vi "StopAcqusition1.vi"(8 "error in (no error)":errorcluster, 11 "Camera_Prime95B in":refnum<class "Camera_Prime95B.lvclass">) -> (0 "error out":errorcluster, 3 "Camera_Prime95B out":refnum<class "Camera_Prime95B.lvclass">)   [LabVIEW 2020]
uses:
  Camera_Prime95B.lvclass
  E:/Development/DevHardSoftware/MicroscopyFramework/Model/Hardware Layer/Real Hardware/Camera_Prime95B/Camera_Prime95B/Dependencies/PVCamNET.dll
  Dependencies/PVCamNET.dll
  Hardware Abstraction Layer/Component/Device/Device/DeviceStatus.ctl
  Hardware Abstraction Layer/Component/Device/Device.lvlib
  E:/Development/DevHardSoftware/MicroscopyFramework/Model/Hardware Abstraction Layer/Component/Camera/Camera/Camera.lvclass
  E:/Development/DevHardSoftware/MicroscopyFramework/Model/Hardware Abstraction Layer/Component/Device/Device/Device.lvclass
  C:/Program Files/National Instruments/LabVIEW 2020/vi.lib/ActorFramework/Actor/Actor.lvclass
  E:/Development/DevHardSoftware/MicroscopyFramework/Model/Hardware Layer/Real Hardware/Camera_Prime95B/Camera_Prime95B/Camera_Prime95B.lvclass
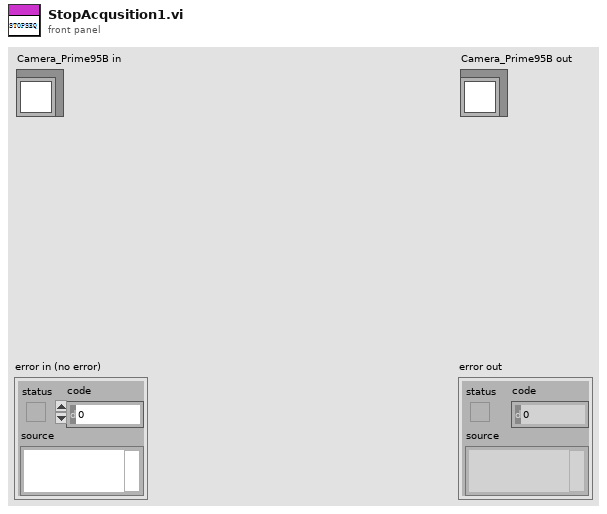
[diagram p1: front panel]
types:
  T1 = typedef "Device.lvlib/DeviceStatus.ctl" = i32
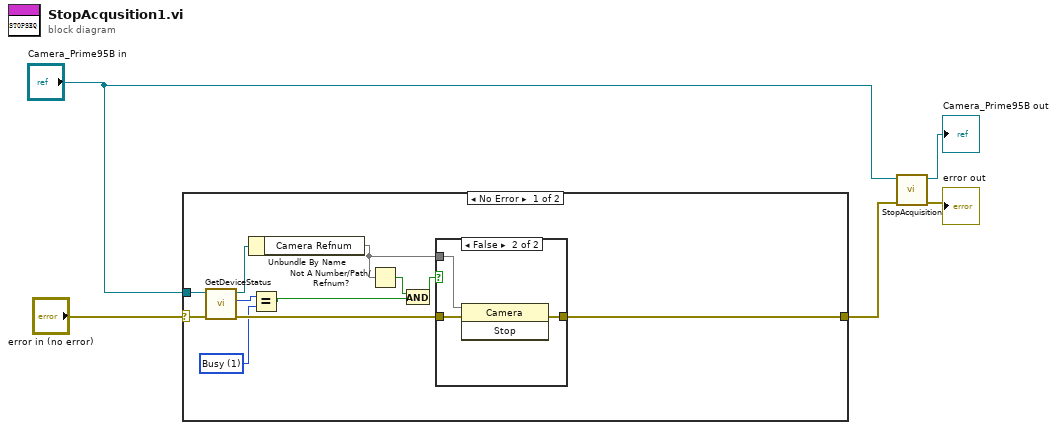
[diagram p0: block diagram]
diagram:
  n1 = case shown="No Error" "error in (no error)" {
    selector: "error in (no error)" -> [w14 w21]
    tunnel: [w16 w21] -> w1
    tunnel: "Camera_Prime95B in" -> [w12 _]
    frame No Error {
      w7 = T1 1 items=["Idle", "Busy"] ("y")
      n2 = call-dynamic "GetDeviceStatus.vi"("error in (no error)"=w14, "Camera_Prime95B in"=w12) -> ("error out"=w13:errorcluster, "Status"=w8:T1, "Camera_Prime95B out"=w11:refnum<class "Camera_Prime95B.lvclass">)  [unwired: 7 in]
      n3 = Unbundle By Name(w11) -> ("Camera Refnum"=w15)
      n4 = Equal?(x=w8, y=w7) -> (x = y?=w6:bool)
      n5 = Not A Number/Path/Refnum?(number/path/refnum=w15) -> (NaN/Path/Refnum?=w10:bool)
      n6 = And(x=w10, y=w6) -> (x .and. y?=w9:bool)
      n7 = case shown="False" w9 {
        tunnel: [w17 w20] -> w16
        tunnel: w13 -> [w17 w19]
        tunnel: w15 -> [_ w18]
        frame True {
        }
        frame False {
          n8 = invoke class="Camera" method="Stop"(reference=w18, error in=w19) -> (error out=w20:errorcluster)  [unwired: 1 in, 2 out]
        }
      }
    }
    frame Error {
    }
  }
  n9 = call-dynamic "StopAcquisition.vi"("error in (no error)"=w1, "Camera_Prime95B in"="Camera_Prime95B in") -> ("error out"=→"error out":errorcluster, "Camera_Prime95B out"=→"Camera_Prime95B out":refnum<class "Camera_Prime95B.lvclass">)  [unwired: 8 in]
